vi "Trim Input JSON (and null).vi"(11 "JSON Input":string) -> (3 "<JSON>":string)   [LabVIEW 2019, in "JSONtext.lvlib"]
uses:
  JSONtext.lvlib
  JDP Science Common Utilities/JDP Utility.lvlib
panel:
  # "Make empty input count as null"
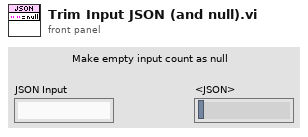
[diagram p1: front panel]
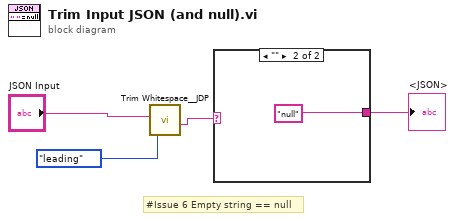
[diagram p0: block diagram]
diagram:
  # "#Issue 6 Empty string == null"
  n1 = call "Trim Whitespace__JDP.vi"("Remove (leading and trailing)"=enum16{"leading", "trailing", "both"}."leading", "String in"="JSON Input") -> ("String out"=w3:string)  [unwired: 5 in]
  n2 = case shown="\"\"" w3 {
    selector: w3 -> [w5 _]
    tunnel: [w5 "null"] -> w2
    frame Default {
    }
    frame "" {
    }
  }
  "<JSON>" <- w2
